vi "poly_control_signalling_write_caller_single.vi"(6 "mode (Sgnl)":T1(ring)=enum."Val(Sgnl)", 8 "error in (no error)":errorcluster, 9 "Value":variant, 10 "Control Name":string, 11 "name of caller in (your caller)":string) -> (0 "error out":errorcluster, 2 "controll reference out":refnum<vi>, 4 "found?":bool)   [LabVIEW 2015]
uses:
  poly_ref_tools_eco_plus.vi
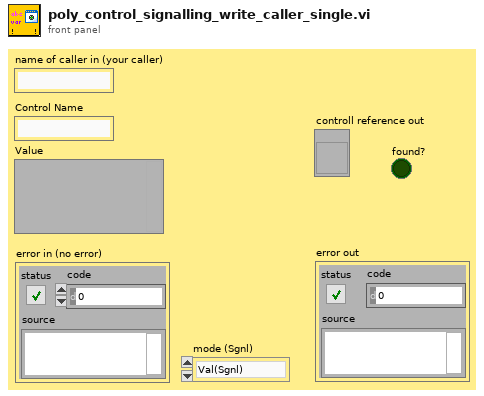
[diagram p1: front panel]
types:
  T1 = enum16{"Val", "Val(Sgnl)", "Val(Undo)", "Method"}
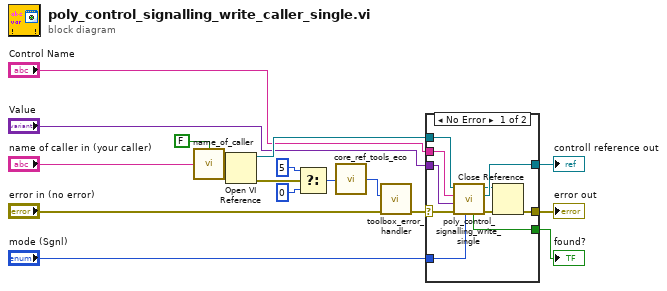
[diagram p0: block diagram]
diagram:
  n1 = call "name_of_caller.vi"("is in inlined vi? (F)"=FALSE, "name of caller in"="name of caller in (your caller)") -> ("name of caller out"=w16:string)  [unwired: 2 in]
  n2 = Open VI Reference(vi path=w16) -> (vi reference=w15:refnum<vi>, error out=w3:errorcluster)  [unwired: 5 in]
  n3 = Select(t=5, s=w3, f=0) -> (s? t:f=w5:i32)
  n4 = call-poly "core_ref_tools_eco.vi"("code (w/out eco)"=w5) -> ("code (+ eco)"=w4:i32)  [unwired: 4 in]
  n5 = call "toolbox_error_handler.vi"("error in (no error)"="error in (no error)", "code (0 = no error)"=w4) -> ("error out"=w1:errorcluster)  [unwired: 8 in, 1 out]
  n6 = case shown="No Error" w1 {
    selector: w1 -> [w18 w28]
    tunnel: w15 -> [w27 _]
    tunnel: "Control Name" -> [w26 _]
    tunnel: "Value" -> [w25 _]
    tunnel: "mode (Sgnl)" -> [w24 _]
    tunnel: [w23 _] -> w11
    tunnel: [w22 _] -> w10
    tunnel: [w19 w28] -> w9
    frame No Error {
      n7 = call "poly_control_signalling_write_single.vi"("mode (Sgnl)"=w24, "error in (no error)"=w18, "Value"=w25, "Control Name"=w26, "vi ref in"=w27) -> ("error out"=w20:errorcluster, "controll reference out"=w22:refnum<vi>, "vi ref out"=w21:refnum<vi>, "found?"=w23:bool)  [unwired: 3 in]
      n8 = Close Reference(reference=w21, error in (no error)=w20) -> (error out=w19:errorcluster)
    }
    frame Error {
    }
  }
  "error out" <- w9
  "controll reference out" <- w10
  "found?" <- w11
